vi "Read Buffer Size.vi"(8 "error in (no error)":errorcluster, 11 "2D U16 DVR Array in":refnum<class "2D U16 DVR Array.lvclass">) -> (0 "error out":errorcluster, 2 "Buffer Size":i32, 3 "2D U16 DVR Array out":refnum<class "2D U16 DVR Array.lvclass">)   [LabVIEW 2024, in "2D U16 DVR Array.lvclass"]
uses:
  2D U16 DVR Array.lvclass
  2D U16 DVR Array.lvclass/2D U16 DVR Array.ctl
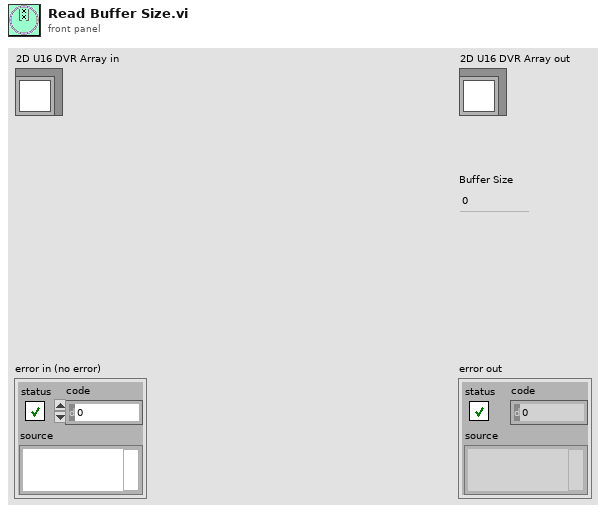
[diagram p1: front panel]
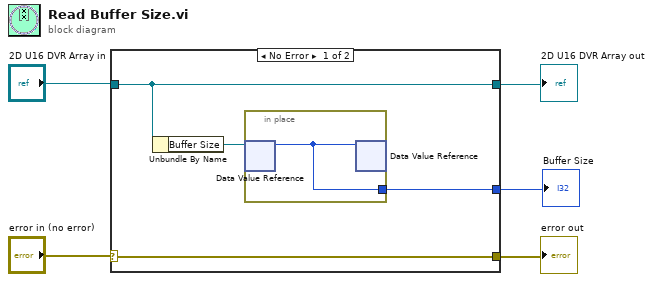
[diagram p0: block diagram]
diagram:
  n1 = case shown="No Error" "error in (no error)" {
    selector: "error in (no error)" -> [w9 w11]
    tunnel: [w9 w11] -> w2
    tunnel: [w8 w12] -> w4
    tunnel: "2D U16 DVR Array in" -> [w8 w12]
    tunnel: [w6 _] -> w1
    frame No Error {
      n2 = Unbundle By Name(w8) -> ("Buffer Size"=w7:refnum<data-value>)
      n3 = in-place {
        in-place-border: [w10] -> w6
        n4 = in-place-dvr #1(w7) -> (w10:i32)  [unwired: 1 out]
        n5 = in-place-dvr #1(w10) -> ()  [unwired: 2 out]
      }
    }
    frame Error {
    }
  }
  "error out" <- w2
  "2D U16 DVR Array out" <- w4
  "Buffer Size" <- w1
